vi "Module Type.vi"(11 "ToggleTestModule in":refnum<class "ToggleTestModule.lvclass">) -> (2 "Module Type":string)   [LabVIEW 2020, in "VolatusScratch.lvlib" / "ToggleTestModule.lvclass"]
uses:
  ToggleTestModule.lvclass
  ToggleTestModule.lvclass/ToggleTestModule.ctl
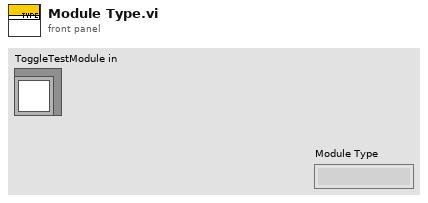
[diagram p1: front panel]
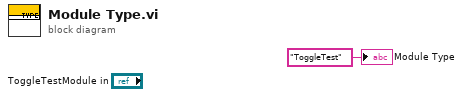
[diagram p0: block diagram]
diagram:
  "Module Type" <- "ToggleTest" ("Module Type")
